vi "look_up_database.vi"(8 "error in (no error)":errorcluster, 10 "Label.Text":string, 11 "Refnum in":T1) -> (0 "error out":errorcluster, 1 "Numeric":i32, 2 "String":string, 3 "Refnum out":T1)   [LabVIEW 2015]
uses:
  <vilib>/addons/database/Connection.llb/Conn ObjectReference.ctl
  <vilib>/addons/database/NI_Database_API.lvlib
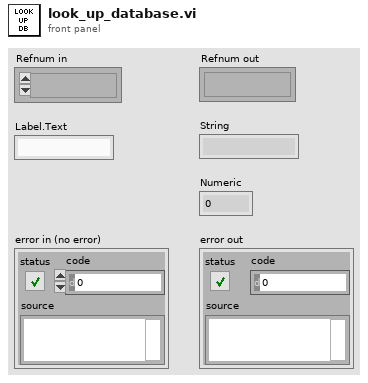
[diagram p1: front panel]
types:
  T1 = typedef "NI_Database_API.lvlib/Conn ObjectReference.ctl" = refnum<k1>
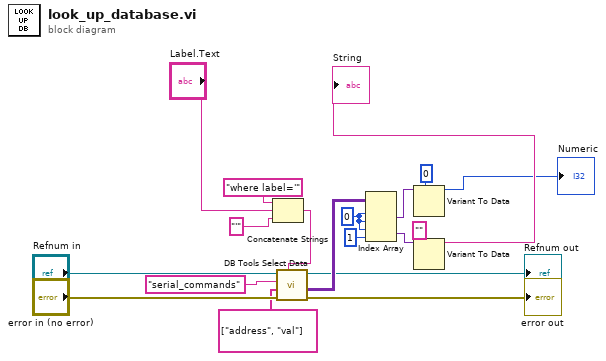
[diagram p0: block diagram]
diagram:
  w12 = 0
  n1 = Concatenate Strings("where label='" ("condition"), "Label.Text", "'") -> (w8:string)
  n2 = call <vilib>:"DB Tools Select Data.vi"("condition"=w8, "error in (no error)"="error in (no error)", "columns"=string[] ["address", "val"], "table"="serial_commands", "connection reference"="Refnum in") -> ("error out"=→"error out":errorcluster, "data"=w11:variant[][], "connection reference out"=→"Refnum out":T1)  [unwired: 1 in]
  n3 = Index Array(array=w11, index (row) #1=w12, index (col) #1=w12, index (row) #2=w12, index (col) #2=1 ("disabled index (col)")) -> (element #1=w14:variant, element #2=w16:variant)
  n4 = Variant To Data(type=0, Variant=w14) -> (data=→"Numeric":i32)  [unwired: 1 in, 1 out]
  n5 = Variant To Data(type="", Variant=w16) -> (data=→"String":string)  [unwired: 1 in, 1 out]
